vi "Instrument_Create.vi"(8 "Error In":errorcluster, 10 "IConfigure":refnum<class "IConfigure.lvclass">, 11 "reference in":refnum<class "Instrument.lvclass">) -> (0 "Error Out":errorcluster, 3 "reference out":refnum<class "Instrument.lvclass">)   [LabVIEW 2023, in "HAL GOOP4.lvlib" / "Instrument.lvclass"]
uses:
  Instrument.lvclass
  Interfaces/IConfigure/IConfigure.lvclass
  Instrument.lvclass/Instrument.ctl
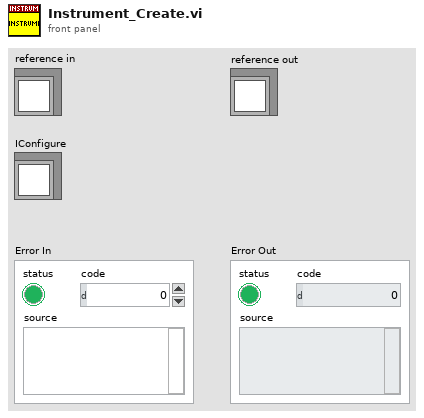
[diagram p1: front panel]
types:
  T1 = typedef "HAL GOOP4.lvlib/Instrument.lvclass/ObjectAttributes.ctl" = cluster{"IConfigure":refnum<class "IConfigure.lvclass">, "Ref Count":u8, "Start Count":u8}
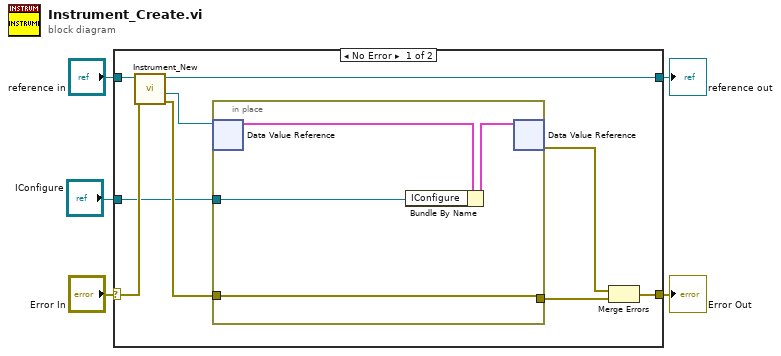
[diagram p0: block diagram]
diagram:
  n1 = case shown="No Error" "Error In" {
    selector: "Error In" -> [w13 w20]
    tunnel: [w11 w20] -> w4
    tunnel: "reference in" -> [w14 w19]
    tunnel: [w8 w19] -> w2
    tunnel: "IConfigure" -> [w6 _]
    frame No Error {
      n2 = call "Instrument_New.vi"("Error In"=w13, "reference in"=w14) -> ("Error Out"=w7:errorcluster, "DVRRefOut"=w10:refnum<data-value>, "reference out"=w8:refnum<class "Instrument.lvclass">)  [unwired: 6 in, 1 out]
      n3 = in-place {
        in-place-border: [w16] -> w12
        in-place-border: w7 -> [w16]
        in-place-border: w6 -> [w15]
        n4 = in-place-dvr #1(w10) -> (w18:T1)  [unwired: 1 out]
        n5 = Bundle By Name(cluster=w18, "IConfigure"=w15) -> (w17:T1)
        n6 = in-place-dvr #1(w17) -> (w9:errorcluster)  [unwired: 1 out]
      }
      n7 = Merge Errors(w9, w12) -> (w11:errorcluster)
    }
    frame Error {
      # "VI-TechBaseTemplate_Simple_4x4x4"
    }
  }
  "Error Out" <- w4
  "reference out" <- w2
